vi "verify table.vi"() -> ()   [LabVIEW 2019, in "Calibration Lib.lvlib"]
uses:
  Calibration Lib.lvlib
  <vilib>/Utility/miscctls.llb/LVRowAndColumnTypeDef.ctl
  <vilib>/Utility/NIReport.llb/Report Type.ctl
  <vilib>/addons/_office/_exclsub.llb/font.ctl
  <vilib>/addons/database/Connection.llb/DB Tools Open Connec (String).vi
  <vilib>/addons/_office/excel.llb/Excel Easy Table (str).vi
  database.lvlib
  <vilib>/addons/_office/NI_ReportGenerationToolkit.lvlib
  <vilib>/Utility/NIReport.llb/NI_report.lvclass
  <vilib>/Utility/NIReport.llb/NI_ReportGenerationCore.lvlib
  <vilib>/addons/database/NI_Database_API.lvlib
panel:
  out "Error out":errorcluster
  out "error out":errorcluster
  in  "Save":bool
  in  "16mm<":dbl format="%.2f"
  in  "14-16mm":dbl format="%.2f"
  in  "12.7-14mm":dbl format="%.2f"
  in  "11-12.7mm":dbl format="%.2f"
  in  "9.5-11mm":dbl format="%.2f"
  in  "8-9.5mm":dbl format="%.2f"
  in  "6.3-8mm":dbl format="%.2f"
  in  "<6.3mm":dbl format="%.2f"
  out "Error out 2":errorcluster
  out "data":string[][](array[string])
  in  "Disc Number":string(combo)
  out "Calibration String":string
  in  "Close":bool
  out "Verify Table":string[][](table)
  # "Labratory Result"
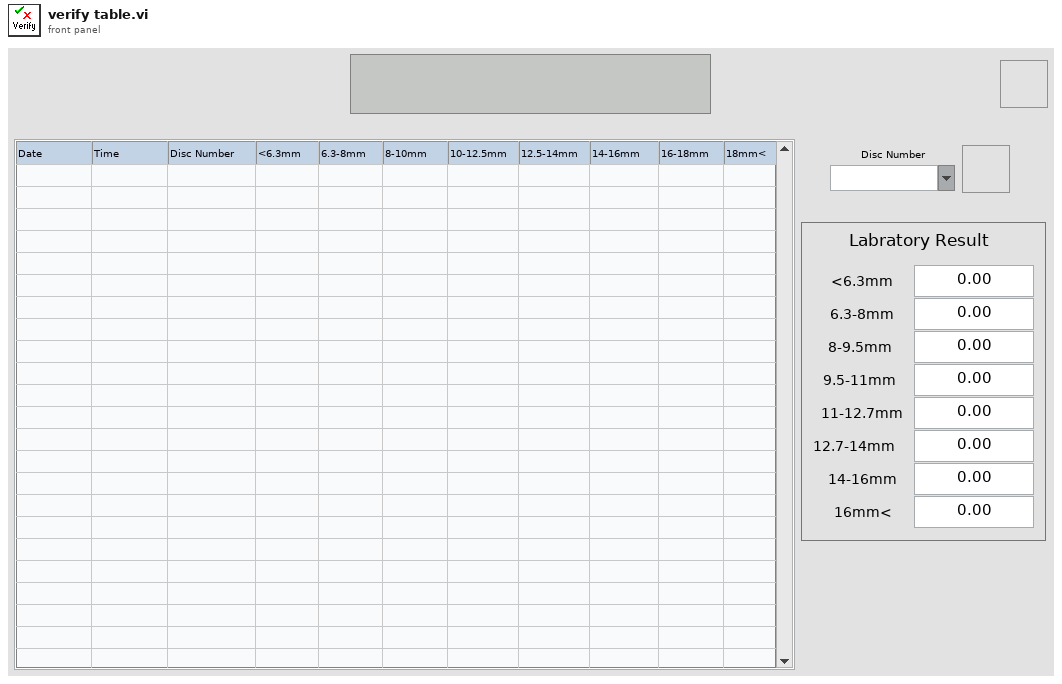
[diagram p1: front panel]
types:
  T1 = typedef "LVRowAndColumnTypeDef.ctl" = cluster{"Row":i32, "Column":i32}
  T2 = enum16{"None", "On Hover", "On Key Focus", "On Hover or Key Focus"}
  T3 = typedef "NI_ReportGenerationToolkit.lvlib/font.ctl" = cluster{"font name":string, "font size":dbl, "bold":u16, "italic":u16, "underline":u16, "strike through":u16, "font color":u32}
  T4 = typedef "NI_ReportGenerationCore.lvlib/Report Type.ctl" = enum16{"HTML", "Word", "Excel"}
  T5 = enum16{"maximized", "minimized", "normal", "no change"}
  T6 = cluster{"date/time string":string, "date/time string":string, "Value":string, "<6.3mm":dbl, "6.3-8mm":dbl, "8-9.5mm":dbl, "9.5-11mm":dbl, "11-12.7mm":dbl, "12.7-14mm":dbl, "14-16mm":dbl, "16mm<":dbl}
  T7 = typedef "NI_Database_API.lvlib/Conn ObjectReference.ctl" = refnum<k1>
  T8 = cluster{i32, "date/time string":string, "date/time string":string, "Value":string, "<6.3mm":dbl, "6.3-8mm":dbl, "8-9.5mm":dbl, "9.5-11mm":dbl, "11-12.7mm":dbl, "12.7-14mm":dbl, "14-16mm":dbl, "16mm<":dbl, dbl, dbl, dbl, dbl, dbl, dbl, dbl, dbl}
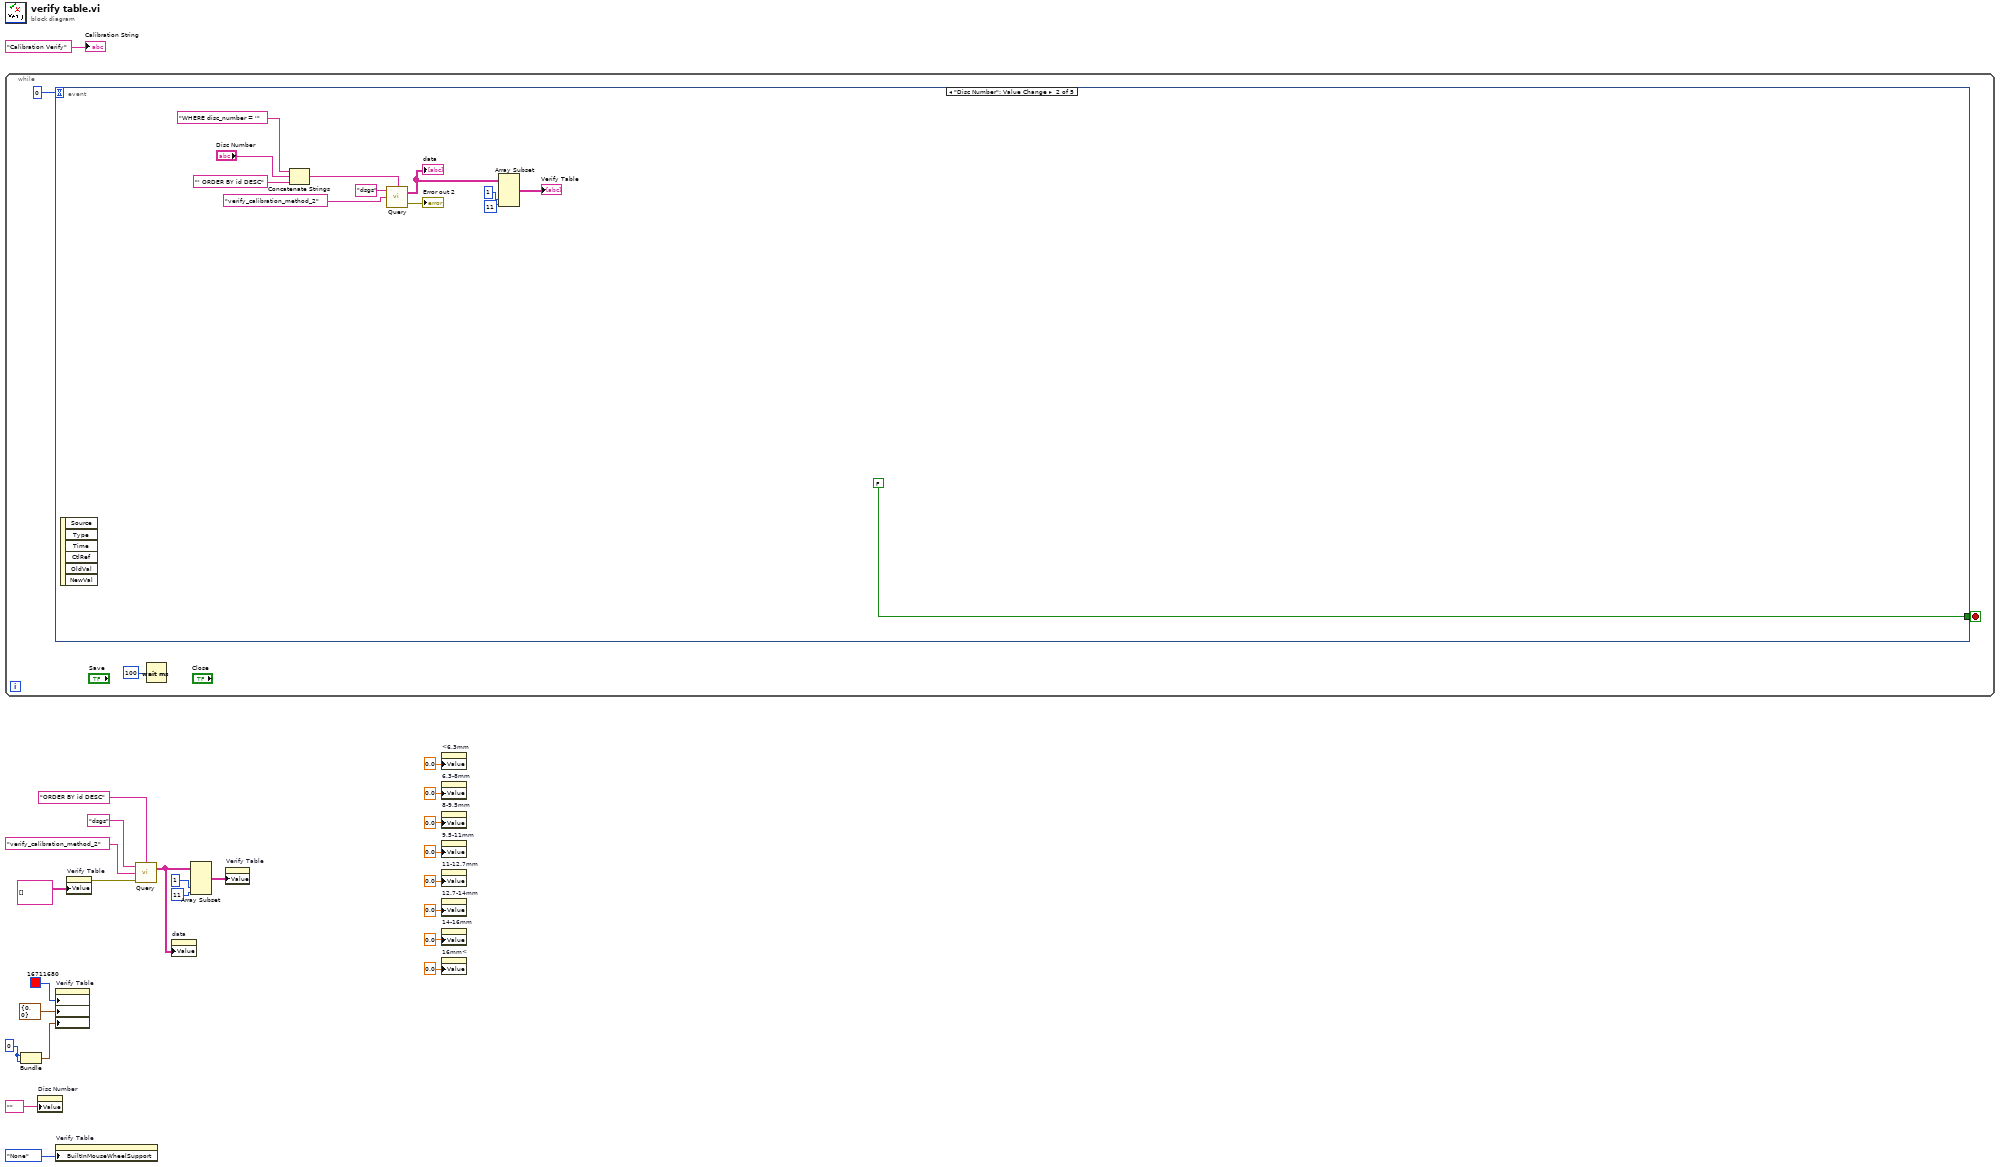
[diagram p0: block diagram]
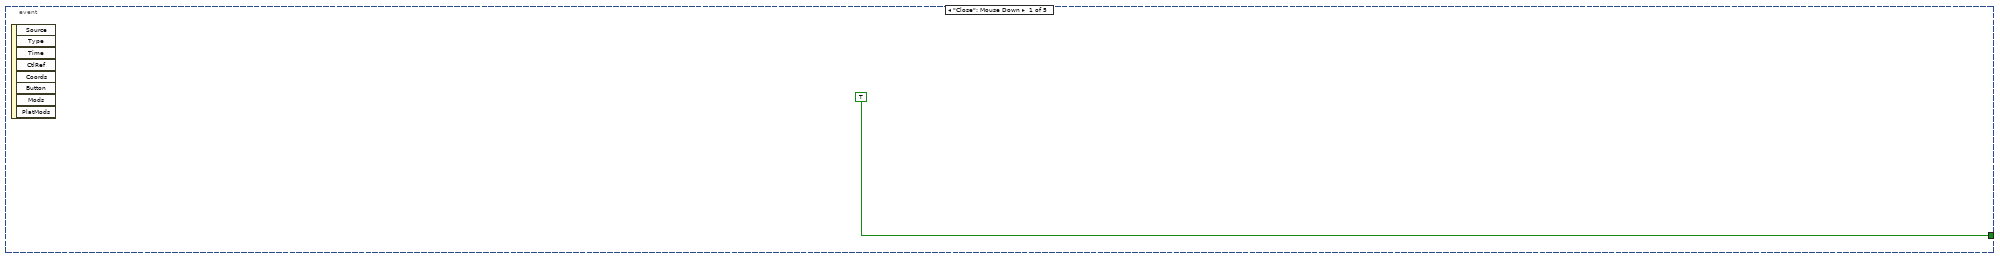
[diagram p2: hidden frame]
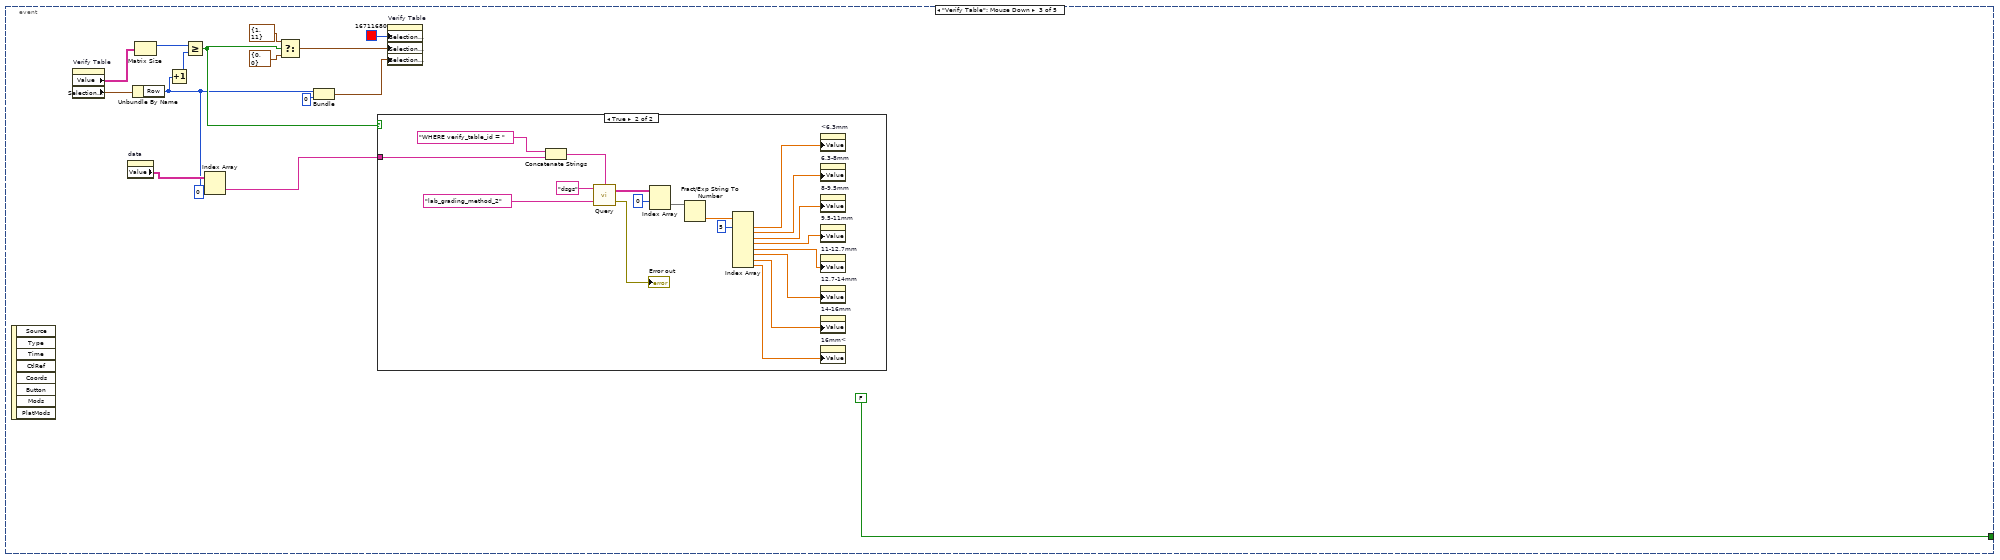
[diagram p3: hidden frame]
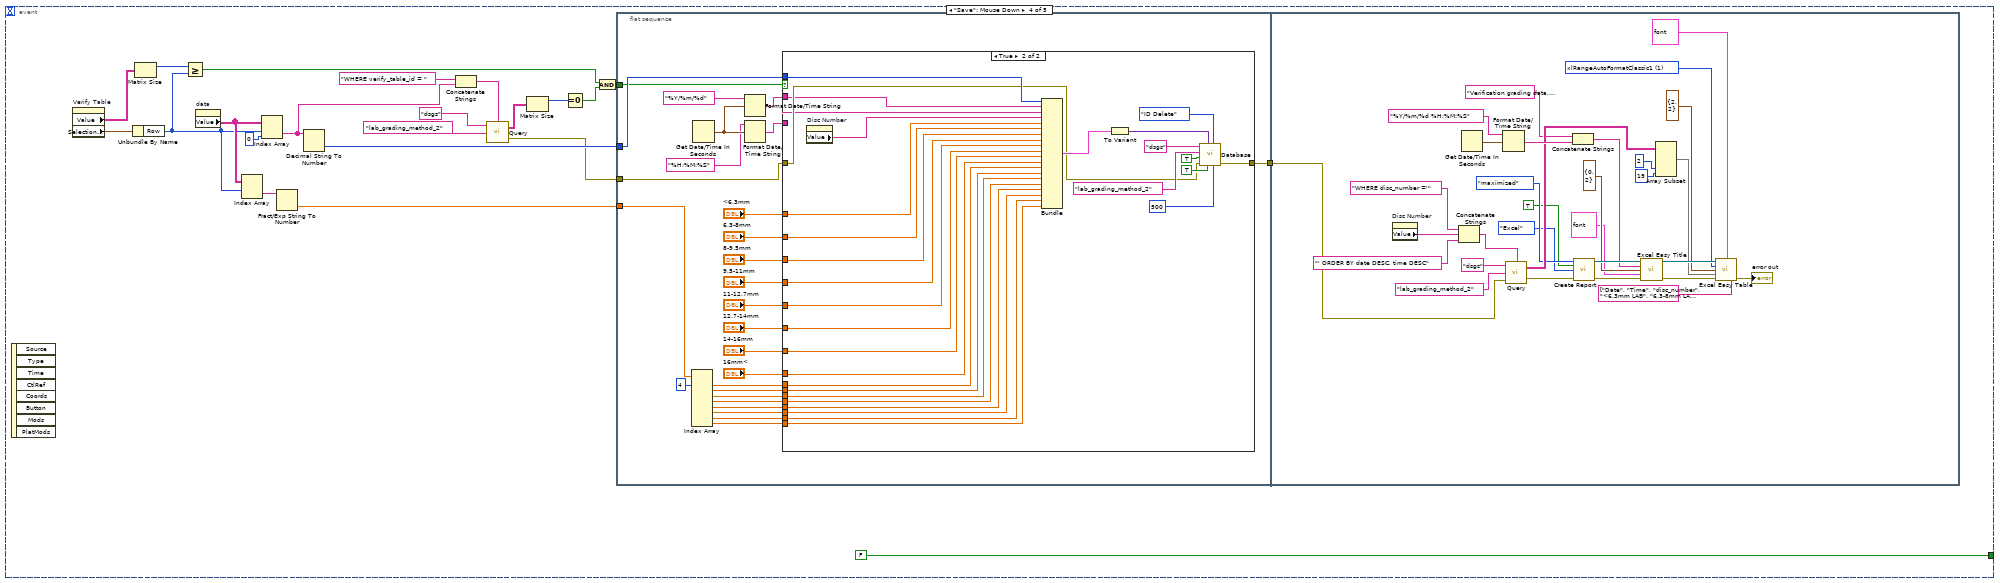
[diagram p5: hidden frame]
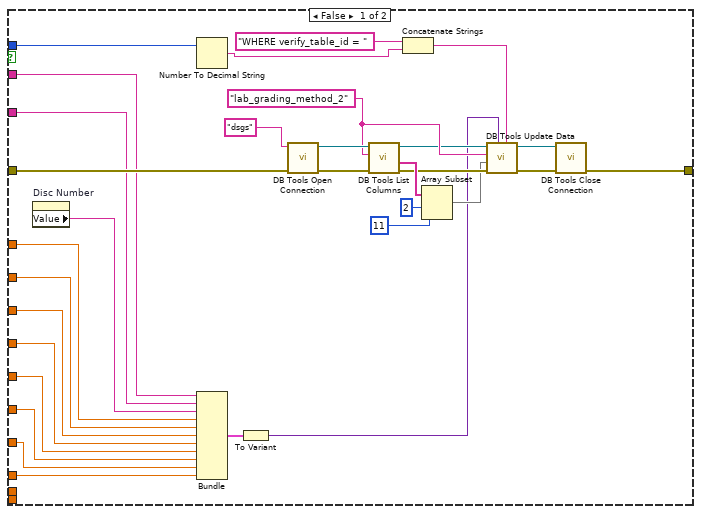
[diagram p6: hidden frame]
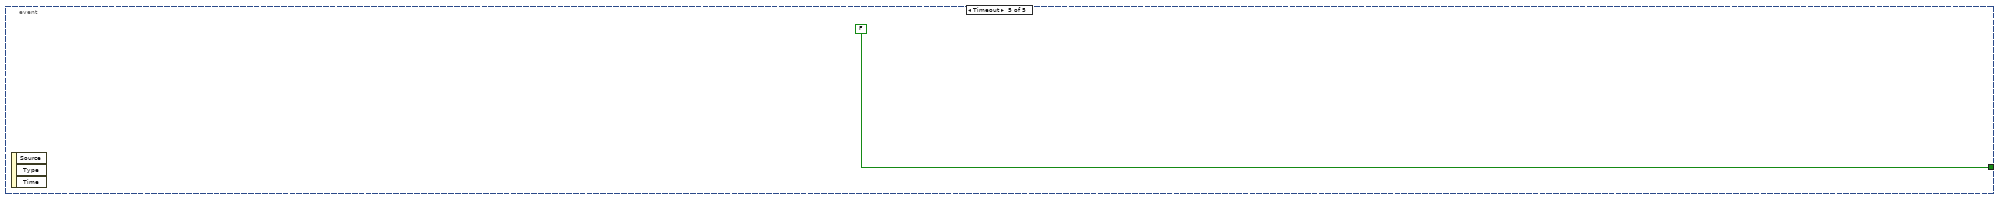
[diagram p7: hidden frame]
diagram:
  w11 = 0 ("Row")
  n1 = while {
    stop <- w26 stop-if-true
    n2 = event shown="[1] \"Disc Number\": Value Change" {
      selector: _ -> [_ _ _ _ _]
      dyn-events: _ -> [_ _ _ _ _]
      timeout: 0 -> [_ _ _ _ _]
      tunnel: [TRUE FALSE FALSE FALSE FALSE] -> w26
      event "Close": Mouse Down {
        n3 = event-data() -> ()  [unwired: 1 in, 8 out]
      }
      event "Disc Number": Value Change {
        n4 = event-data() -> ()  [unwired: 1 in, 6 out]
        n5 = Concatenate Strings("WHERE disc_number = '" ("string"), "Disc Number", "' ORDER BY id DESC" ("string")) -> (w35:string)
        n6 = call "Query.vi"("Condition"=w35, "Table Name"="verify_calibration_method_2", "Connection Name"="dsgs") -> ("Error out"=→"Error out 2":errorcluster, "data"=w30:string[][])  [unwired: 1 in]
        "data" <- w30
        n7 = Array Subset(array=w30, index (col)=1 ("index"), length (col)=11 ("length")) -> (→"Verify Table":string[][])  [unwired: 2 in]
      }
      event "Verify Table": Mouse Down {
        n8 = event-data() -> ()  [unwired: 1 in, 8 out]
        n9 = property on="Verify Table" class="Tbl (strict)"() -> ("Value"=w51:string[][], "Selection Start"=w55:T1)  [unwired: 2 in, 2 out]
        n10 = property on="data" class="Arr (strict)"() -> ("Value"=w45:string[][])  [unwired: 2 in, 2 out]
        n11 = Unbundle By Name(w55) -> ("Row"=w42:i32)
        n12 = Matrix Size(0:w51) -> (1:w50:i32)  [unwired: 1 out]
        n13 = Increment(x=w42) -> (x+1=w41:i32)
        n14 = Greater Or Equal?(x=w50, y=w41) -> (x >= y?=w46:bool)
        n15 = Index Array(array=w45, index (row)=w42, index (col)=0 ("disabled index (col)")) -> (element=w43:string)
        n16 = Select(t=T1 {"Row"=1, "Column"=11} ("Selection Size"), s=w46, f=T1 {"Row"=0, "Column"=0}) -> (s? t:f=w48:T1)
        n17 = Bundle("Row"=w42, "Row"=0) -> (w52:cluster{"Row":i32, "Row":i32})  [unwired: 1 in]
        n18 = case shown="True" w46 {
          tunnel: w43 -> [_ w71]
          frame False {
          }
          frame True {
            n19 = Concatenate Strings("WHERE verify_table_id = " ("string"), w71) -> (w75:string)
            n20 = call "Query.vi"("Condition"=w75, "Table Name"="lab_grading_method_2", "Connection Name"="dsgs") -> ("Error out"=→"Error out":errorcluster, "data"=w70:string[][])  [unwired: 1 in]
            n21 = Index Array(array=w70, index (row)=0) -> (element=w67:string[])  [unwired: 1 in]
            n22 = Fract/Exp String To Number(string=w67) -> (number=w66:dbl[])  [unwired: 3 in, 1 out]
            n23 = Index Array(array=w66, index #1=5 ("index")) -> (element #1=w61:dbl, element #2=w62:dbl, element #3=w63:dbl, element #4=w65:dbl, element #5=w64:dbl, element #6=w58:dbl, element #7=w59:dbl, element #8=w60:dbl)  [unwired: 7 in]
            n24 = property on="<6.3mm" class="DigNum (strict)"("Value"=w61) -> ()  [unwired: 2 in, 2 out]
            n25 = property on="6.3-8mm" class="DigNum (strict)"("Value"=w62) -> ()  [unwired: 2 in, 2 out]
            n26 = property on="8-9.5mm" class="DigNum (strict)"("Value"=w63) -> ()  [unwired: 2 in, 2 out]
            n27 = property on="9.5-11mm" class="DigNum (strict)"("Value"=w65) -> ()  [unwired: 2 in, 2 out]
            n28 = property on="11-12.7mm" class="DigNum (strict)"("Value"=w64) -> ()  [unwired: 2 in, 2 out]
            n29 = property on="12.7-14mm" class="DigNum (strict)"("Value"=w58) -> ()  [unwired: 2 in, 2 out]
            n30 = property on="14-16mm" class="DigNum (strict)"("Value"=w59) -> ()  [unwired: 2 in, 2 out]
            n31 = property on="16mm<" class="DigNum (strict)"("Value"=w60) -> ()  [unwired: 2 in, 2 out]
          }
        }
        n32 = property on="Verify Table" class="Tbl (strict)"("Selection Color"=u32 16711680, "Selection Size"=w48, "Selection Start"=w52) -> ()  [unwired: 2 in, 2 out]
      }
      event "Save": Mouse Down {
        n33 = event-data() -> ()  [unwired: 1 in, 8 out]
        n34 = property on="Verify Table" class="Tbl (strict)"() -> ("Value"=w96:string[][], "Selection Start"=w97:T1)  [unwired: 2 in, 2 out]
        n35 = Unbundle By Name(w97) -> ("Row"=w90:i32)
        n36 = Matrix Size(0:w96) -> (1:w95:i32)  [unwired: 1 out]
        n37 = Greater Or Equal?(x=w95, y=w90) -> (x >= y?=w80:bool)
        n38 = property on="data" class="Arr (strict)"() -> ("Value"=w91:string[][])  [unwired: 2 in, 2 out]
        n39 = Index Array(array=w91, index (row)=w90) -> (element=w89:string[])  [unwired: 1 in]
        n40 = Index Array(array=w91, index (row)=w90, index (col)=0 ("disabled index (col)")) -> (element=w83:string)
        n41 = Fract/Exp String To Number(string=w89) -> (number=w88:dbl[])  [unwired: 3 in, 1 out]
        n42 = Decimal String To Number(string=w83) -> (number=w92:i32)  [unwired: 2 in, 1 out]
        n43 = Concatenate Strings("WHERE verify_table_id = " ("string"), w83) -> (w84:string)
        n44 = call "Query.vi"("Condition"=w84, "Table Name"="lab_grading_method_2", "Connection Name"="dsgs") -> ("Error out"=w77:errorcluster, "data"=w82:string[][])  [unwired: 1 in]
        n45 = Matrix Size(0:w82) -> (1:w81:i32)  [unwired: 1 out]
        n46 = Equal To 0?(x=w81) -> (x = 0?=w78:bool)
        n47 = And(x=w80, y=w78) -> (x .and. y?=w79:bool)
        n48 = flat-sequence {
          tunnel: w92 -> [w124]
          tunnel: w88 -> [w119]
          tunnel: w79 -> [w123]
          tunnel: w77 -> [w122]
          tunnel: [w121] -> w76
          tunnel: w76 -> [w186]
          frame #0 {
            n49 = Index Array(array=w119, index #1=4 ("index")) -> (element #1=w118:dbl, element #2=w111:dbl, element #3=w112:dbl, element #4=w113:dbl, element #5=w114:dbl, element #6=w115:dbl, element #7=w116:dbl, element #8=w117:dbl)  [unwired: 7 in]
            n50 = Get Date/Time In Seconds() -> (seconds since 1Jan1904=w110:timestamp)
            n51 = Format Date/Time String(time format string (%c)="%Y/%m/%d", seconds (now)=w110) -> (date/time string=w107:string)  [unwired: 1 in]
            n52 = Format Date/Time String(time format string (%c)="%H:%M:%S", seconds (now)=w110) -> (date/time string=w106:string)  [unwired: 1 in]
            n53 = case shown="True" w123 {
              tunnel: w124 -> [w127 w180]
              tunnel: w122 -> [w155 w175]
              tunnel: [w129 w174] -> w121
              tunnel: w118 -> [_ w173]
              tunnel: w117 -> [_ w172]
              tunnel: w116 -> [_ w171]
              tunnel: w115 -> [_ w170]
              tunnel: w114 -> [_ w169]
              tunnel: w113 -> [_ w168]
              tunnel: w112 -> [_ w167]
              tunnel: w111 -> [_ w166]
              tunnel: w107 -> [w138 w165]
              tunnel: w106 -> [w139 w164]
              tunnel: "<6.3mm" -> [w141 w163]
              tunnel: "6.3-8mm" -> [w142 w162]
              tunnel: "16mm<" -> [w148 w161]
              tunnel: "14-16mm" -> [w147 w160]
              tunnel: "12.7-14mm" -> [w146 w159]
              tunnel: "11-12.7mm" -> [w145 w158]
              tunnel: "9.5-11mm" -> [w144 w157]
              tunnel: "8-9.5mm" -> [w143 w156]
              frame False {
                w134 = "lab_grading_method_2" ("table")
                n54 = property on="Disc Number" class="CmbBox"() -> ("Value"=w140:string)  [unwired: 2 in, 2 out]
                n55 = Number To Decimal String(number=w127) -> (decimal integer string=w126:string)  [unwired: 1 in]
                n56 = Bundle("date/time string"=w138, "date/time string"=w139, "Value"=w140, "<6.3mm"=w141, "6.3-8mm"=w142, "8-9.5mm"=w143, "9.5-11mm"=w144, "11-12.7mm"=w145, "12.7-14mm"=w146, "14-16mm"=w147, "16mm<"=w148) -> (w137:T6)  [unwired: 1 in]
                n57 = To Variant(anything=w137) -> (Variant=w132:variant)
                n58 = call-poly <vilib>:"DB Tools Open Connection.vi"("error in (no error)"=w155, "connection information"="dsgs" ("date/time string")) -> ("error out"=w152:errorcluster, "connection reference"=w153:T7)  [unwired: 6 in]
                n59 = call <vilib>:"DB Tools List Columns.vi"("error in (no error)"=w152, "table"=w134, "connection reference"=w153) -> ("error out"=w136:errorcluster, "columns"=w151:string[], "connection reference out"=w133:T7)  [unwired: 1 in, 1 out]
                n60 = Concatenate Strings("WHERE verify_table_id = " ("string"), w126) -> (w125:string)
                n61 = Array Subset(array=w151, index=2, length=11) -> (w135:string[])
                n62 = call <vilib>:"DB Tools Update Data.vi"("condition"=w125, "data"=w132, "error in (no error)"=w136, "columns"=w135, "table"=w134, "connection reference"=w133) -> ("error out"=w131:errorcluster, "connection reference out"=w130:T7)  [unwired: 4 in]
                n63 = call <vilib>:"DB Tools Close Connection.vi"("error in (no error)"=w131, "connection reference"=w130) -> ("error out"=w129:errorcluster)  [unwired: 5 in]
              }
              frame True {
                n64 = property on="Disc Number" class="CmbBox"() -> ("Value"=w181:string)  [unwired: 2 in, 2 out]
                n65 = Bundle(w180, "date/time string"=w165, "date/time string"=w164, "Value"=w181, "<6.3mm"=w163, "6.3-8mm"=w162, "8-9.5mm"=w156, "9.5-11mm"=w157, "11-12.7mm"=w158, "12.7-14mm"=w159, "14-16mm"=w160, "16mm<"=w161, w173, w166, w167, w168, w169, w170, w171, w172) -> (w178:T8)  [unwired: 1 in]
                n66 = To Variant(anything=w178) -> (Variant=w179:variant)
                n67 = call "Database.vi"("Maximum Row"=500, "Enum"=enum16{"ID Delete", "Time Delete"}."ID Delete", "Delete row?"=TRUE, "Data"=w179, "Error in"=w175, "Auto Increment ID?"=TRUE, "Table"="lab_grading_method_2", "Connection"="dsgs") -> ("Error out"=w174:errorcluster)  [unwired: 3 in]
              }
            }
          }
          frame #1 {
            w193 = 1 items=["xlRangeAutoFormat3DEffects1"=13, "xlRangeAutoFormat3DEffects2"=14, "xlRangeAutoFormatAccounting1"=4, "xlRangeAutoFormatAccounting2"=5, "xlRangeAutoFormatAccounting3"=6, "xlRangeAutoFormatAccounting4"=17, "xlRangeAutoFormatClassic1"=1, "xlRangeAutoFormatClassic2"=2, "xlRangeAutoFormatClassic3"=3, "xlRangeAutoFormatColor1"=7, "xlRangeAutoFormatColor2"=8, "xlRangeAutoFormatColor3"=9, "xlRangeAutoFormatList1"=10, "xlRangeAutoFormatList2"=11, "xlRangeAutoFormatList3"=12, "xlRangeAutoFormatLocalFormat1"=15, "xlRangeAutoFormatLocalFormat2"=16, "xlRangeAutoFormatLocalFormat3"=19, "xlRangeAutoFormatLocalFormat4"=20, "xlRangeAutoFormatReport1"=21, "xlRangeAutoFormatReport2"=22, "xlRangeAutoFormatReport3"=23, "xlRangeAutoFormatReport4"=24, "xlRangeAutoFormatReport5"=25, "xlRangeAutoFormatReport6"=26, "xlRangeAutoFormatReport7"=27, "xlRangeAutoFormatReport8"=28, "xlRangeAutoFormatReport9"=29, "xlRangeAutoFormatReport10"=30, "xlRangeAutoFormatClassicPivotTable"=31, "xlRangeAutoFormatTable1"=32, "xlRangeAutoFormatTable2"=33, "xlRangeAutoFormatTable3"=34, "xlRangeAutoFormatTable4"=35, "xlRangeAutoFormatTable5"=36, "xlRangeAutoFormatTable6"=37, "xlRangeAutoFormatTable7"=38, "xlRangeAutoFormatTable8"=39, "xlRangeAutoFormatTable9"=40, "xlRangeAutoFormatTable10"=41, "xlRangeAutoFormatPTNone"=42, "xlRangeAutoFormatNone"=-4142, "xlRangeAutoFormatSimple"=-4154] ("auto format (none)")
            n68 = property on="Disc Number" class="CmbBox"() -> ("Value"=w216:string)  [unwired: 2 in, 2 out]
            n69 = Concatenate Strings("WHERE disc_number ='" ("string"), w216, "' ORDER BY date DESC, time DESC" ("Condition")) -> (w215:string)
            n70 = Get Date/Time In Seconds() -> (seconds since 1Jan1904=w208:timestamp)
            n71 = Format Date/Time String(time format string (%c)="%Y/%m/%d %H:%M:%S", seconds (now)=w208) -> (date/time string=w209:string)  [unwired: 1 in]
            n72 = call "Query.vi"("Condition"=w215, "Error in"=w186, "Table Name"="lab_grading_method_2", "Connection Name"="dsgs") -> ("Error out"=w207:errorcluster, "data"=w206:string[][])
            n73 = Concatenate Strings("Verification grading data, Report generated at " ("title"), w209) -> (w210:string)
            n74 = call <vilib>:"Create Report.vi"("window state (normal)"=T5."maximized", "display alerts? (F)"=TRUE, "report type"=Report_Type."Excel", "error in (no error)"=w207) -> ("report out"=w212:refnum<class "NI_report.lvclass">, "error out"=w214:errorcluster)  [unwired: 10 in]
            n75 = call <vilib>:"Excel Easy Title.vi"("report in"=w212, "title"=w210, "start (0, 0)"=cluster{"row":i32, "column":i32} {"row"=0, "column"=2}, "font"=T3 {"font name"="Times New Roman", "font size"=24.0, "bold"=1, "italic"=0, "underline"=0, "strike through"=0, "font color"=16777216}, "error in (no error)"=w214) -> ("report out"=w211:refnum<class "NI_report.lvclass">, "error out"=w213:errorcluster)  [unwired: 8 in, 1 out]
            n76 = Array Subset(array=w206, index (col)=2 ("index"), length (col)=19 ("length")) -> (w205:string[][])  [unwired: 2 in]
            n77 = call-poly <vilib>:"Excel Easy Table.vi"("report in"=w211, "font"=T3 {"font name"="Times New Roman", "font size"=12.0, "bold"=0, "italic"=0, "underline"=0, "strike through"=0, "font color"=16777216}, "auto format (none)"=w193, "start (0, 0)"=cluster{"row":i32, "column":i32} {"row"=2, "column"=2}, "text data"=w205, "error in (no error)"=w213, "column headers"=string[] ["Date", "Time", "disc_number", "<6.3mm LAB", "6.3-8mm LAB", "8-10mm LAB", "10-12.5mm LAB", "12.5-14mm LAB", "14-16mm LAB", "16-18mm LAB", "18mm< LAB", "<6.3mm SYS", "6.3-8mm SYS", "8-10mm SYS", "10-12.5mm SYS", "12.5-14mm SYS", "14-16mm SYS", "16-18mm SYS", "18mm< SYS"]) -> ("error out"=→"error out":errorcluster)  [unwired: 4 in, 4 out]
          }
        }
      }
      event Timeout {
        n78 = event-data() -> ()  [unwired: 1 in, 3 out]
      }
    }
    n79 = Wait (ms)(milliseconds to wait=u32 100) -> ()  [unwired: 1 out]
  }
  n80 = Bundle("Row"=w11, "Row"=w11) -> (w10:cluster{"Row":i32, "Row":i32})  [unwired: 1 in]
  n81 = property on="Disc Number" class="CmbBox"("Value"="" ("Disc Number")) -> ()  [unwired: 2 in, 2 out]
  n82 = property on="Verify Table" class="Tbl (strict)"("Selection Color"=u32 16711680, "Selection Size"=T1 {"Row"=0, "Column"=0}, "Selection Start"=w10) -> ()  [unwired: 2 in, 2 out]
  n83 = property on="Verify Table" class="Tbl (strict)"("BuiltInMouseWheelSupport"=T2."None" ("Built-In Mouse Wheel Support")) -> ()  [unwired: 2 in, 2 out]
  n84 = property on="Verify Table" class="Tbl (strict)"("Value"=string[][] [] ("Verify Table")) -> (error out=w13:errorcluster)  [unwired: 2 in, 1 out]
  n85 = call "Query.vi"("Condition"="ORDER BY id DESC", "Error in"=w13, "Table Name"="verify_calibration_method_2", "Connection Name"="dsgs") -> ("data"=w17:string[][])  [unwired: 1 out]
  n86 = property on="data" class="Arr (strict)"("Value"=w17) -> ()  [unwired: 2 in, 2 out]
  n87 = Array Subset(array=w17, index (col)=1 ("index"), length (col)=11 ("length")) -> (w20:string[][])  [unwired: 2 in]
  n88 = property on="Verify Table" class="Tbl (strict)"("Value"=w20) -> ()  [unwired: 2 in, 2 out]
  n89 = property on="<6.3mm" class="DigNum (strict)"("Value"=0.0 ("<6.3mm")) -> ()  [unwired: 2 in, 2 out]
  n90 = property on="6.3-8mm" class="DigNum (strict)"("Value"=0.0 ("6.3-8mm")) -> ()  [unwired: 2 in, 2 out]
  n91 = property on="8-9.5mm" class="DigNum (strict)"("Value"=0.0 ("8-10mm")) -> ()  [unwired: 2 in, 2 out]
  n92 = property on="9.5-11mm" class="DigNum (strict)"("Value"=0.0 ("10-12.5mm")) -> ()  [unwired: 2 in, 2 out]
  n93 = property on="11-12.7mm" class="DigNum (strict)"("Value"=0.0 ("12.5-14mm")) -> ()  [unwired: 2 in, 2 out]
  n94 = property on="12.7-14mm" class="DigNum (strict)"("Value"=0.0 ("14-16mm")) -> ()  [unwired: 2 in, 2 out]
  n95 = property on="14-16mm" class="DigNum (strict)"("Value"=0.0 ("16-18mm")) -> ()  [unwired: 2 in, 2 out]
  n96 = property on="16mm<" class="DigNum (strict)"("Value"=0.0 ("18mm<")) -> ()  [unwired: 2 in, 2 out]
  "Calibration String" <- "Calibration Verify" ("Calibration String")
